vi "Encoder Read Value 1.vi"(8 "error in (no error)":errorcluster, 11 "Encoder in":refnum<class "Encoder.lvclass">) -> (0 "error out":errorcluster, 3 "Numeric":i32)   [LabVIEW 2014]
uses:
  <vilib>/LabVIEW Universal Transcriptor/LabVIEW Universal Transcriptor Rotary Encoder Library/Encoder.lvclass
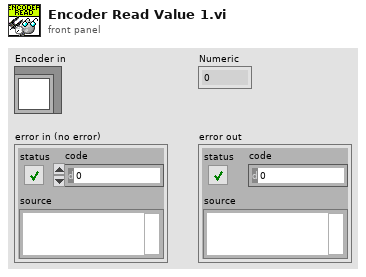
[diagram p1: front panel]
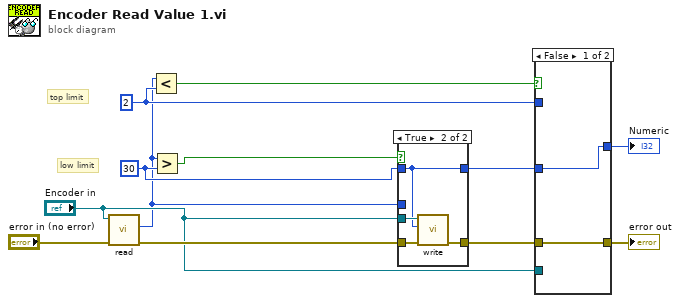
[diagram p0: block diagram]
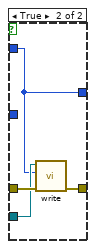
[diagram p2: hidden frame]
diagram:
  w5 = 2 ("y")
  w9 = 30 ("y")
  # "low limit"
  # "top limit"
  n1 = call <vilib>:"read.vi"("error in (no error)"="error in (no error)", "Encoder in"="Encoder in") -> ("error out"=w11:errorcluster, "value"=w1:i32)  [unwired: 7 in]
  n2 = Less?(x=w1, y=w5) -> (x < y?=w8:bool)
  n3 = Greater?(x=w1, y=w9) -> (0:w10:bool)
  n4 = case shown="True" w10 {
    tunnel: w11 -> [w14 w18]
    tunnel: "Encoder in" -> [_ w17]
    tunnel: w9 -> [_ w15]
    tunnel: [w14 w16] -> w7
    tunnel: [w13 w15] -> w4
    tunnel: w1 -> [w13 _]
    frame False {
    }
    frame True {
      n5 = call <vilib>:"write.vi"("error in (no error)"=w18, "value"=w15, "Encoder in"=w17) -> ("error out"=w16:errorcluster)  [unwired: 7 in]
    }
  }
  n6 = case shown="False" w8 {
    tunnel: w7 -> [w20 w24]
    tunnel: "Encoder in" -> [_ w23]
    tunnel: w5 -> [_ w21]
    tunnel: [w20 w22] -> w2
    tunnel: [w19 w21] -> w3
    tunnel: w4 -> [w19 _]
    frame False {
    }
    frame True {
      n7 = call <vilib>:"write.vi"("error in (no error)"=w24, "value"=w21, "Encoder in"=w23) -> ("error out"=w22:errorcluster)  [unwired: 7 in]
    }
  }
  "Numeric" <- w3
  "error out" <- w2
